vi "(SubVI) Calculate Xbd and Xst.vi"(6 "yr":dbl, 7 "cr":dbl, 9 "Stage Position":dbl[](array[numeric]), 10 "QPD signal":dbl[](array[numeric]), 11 "conversion factor (V/um)":dbl) -> (2 "Xst":dbl[](array[numeric]), 3 "Xbd":dbl[](array[numeric]))   [LabVIEW 2014]
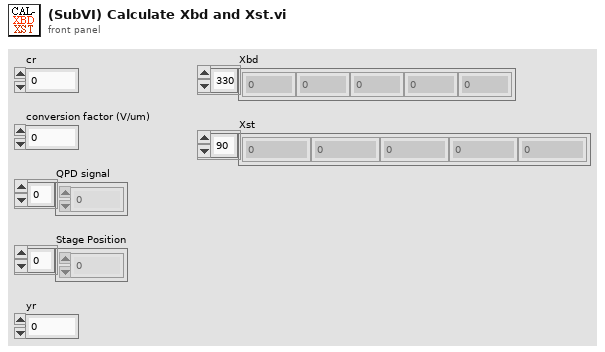
[diagram p1: front panel]
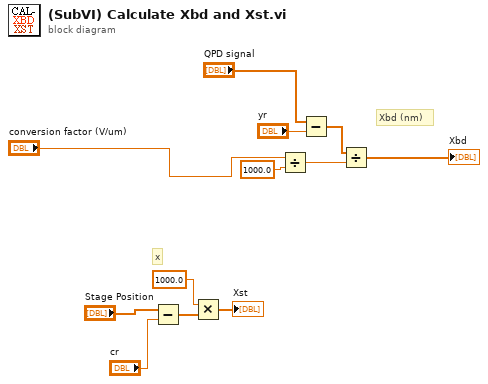
[diagram p0: block diagram]
diagram:
  # "x"
  # "Xbd (nm)"
  n1 = Subtract(x="Stage Position", y="cr") -> (x-y=w3:dbl[])
  n2 = Multiply(x=1000.0, y=w3) -> (x*y=→"Xst":dbl[])
  n3 = Divide(x="conversion factor (V/um)", y=1000.0) -> (x/y=w11:dbl)
  n4 = Subtract(x="QPD signal", y="yr") -> (x-y=w2:dbl[])
  n5 = Divide(x=w2, y=w11) -> (x/y=→"Xbd":dbl[])
